vi "Array-Speedtest.vi"() -> ()   [LabVIEW 2016]
uses:
  <userlib>/_OpenG.lib/lvdata/lvdata.llb/Type Descriptor__ogtk.ctl
  <userlib>/_OpenG.lib/lvdata/lvdata.llb/Type Descriptor Header__ogtk.ctl
  <userlib>/_OpenG.lib/lvdata/lvdata.llb/Type Descriptor Enumeration__ogtk.ctl
  SubVis/msgpack_config.ctl
  SubVis/cluster_conversion.ctl
  SubVis/enum_conversion.ctl
  MsgPack.lvlib
  EncodeTypes/enc_a_I8.vi
  EncodeTypes/enc_a_U16.vi
  EncodeTypes/enc_a_I32.vi
  EncodeTypes/enc_a_U8.vi
  EncodeTypes/enc_a_I64.vi
  EncodeTypes/enc_a_I16.vi
  EncodeTypes/enc_a_U32.vi
  EncodeTypes/enc_a_U64.vi
panel:
  out "Element Type Descriptor":T1
  out "Numeric 4":i32
  out "N dims 2":u32
  out "time 4":u32
  out "Array 2":u32[](array[numeric])
  out "N dims":u32
  out "Size(s)":u32[](array[numeric])
  out "x = y?":bool
  out "ms/iter 2":dbl
  out "ms/iter 3":dbl
  out "Array Out 2":u8[](array[numeric]) format="%.0x"
  out "Array Out":u8[](array[numeric]) format="%.0x"
  out "Numeric 3":i32
  out "time 3":u32
  out "Array":u32[](array[numeric])
  out "Type Descriptor Header 2":T2 {"type" format="%.0x"}
  out "Type Descriptor 2":T1
  out "Numeric 2":i32
  out "Numeric":i32
  out "time 2":u32
  out "time":u32
  out "Array":u8[](array[numeric]) format="%.0x"
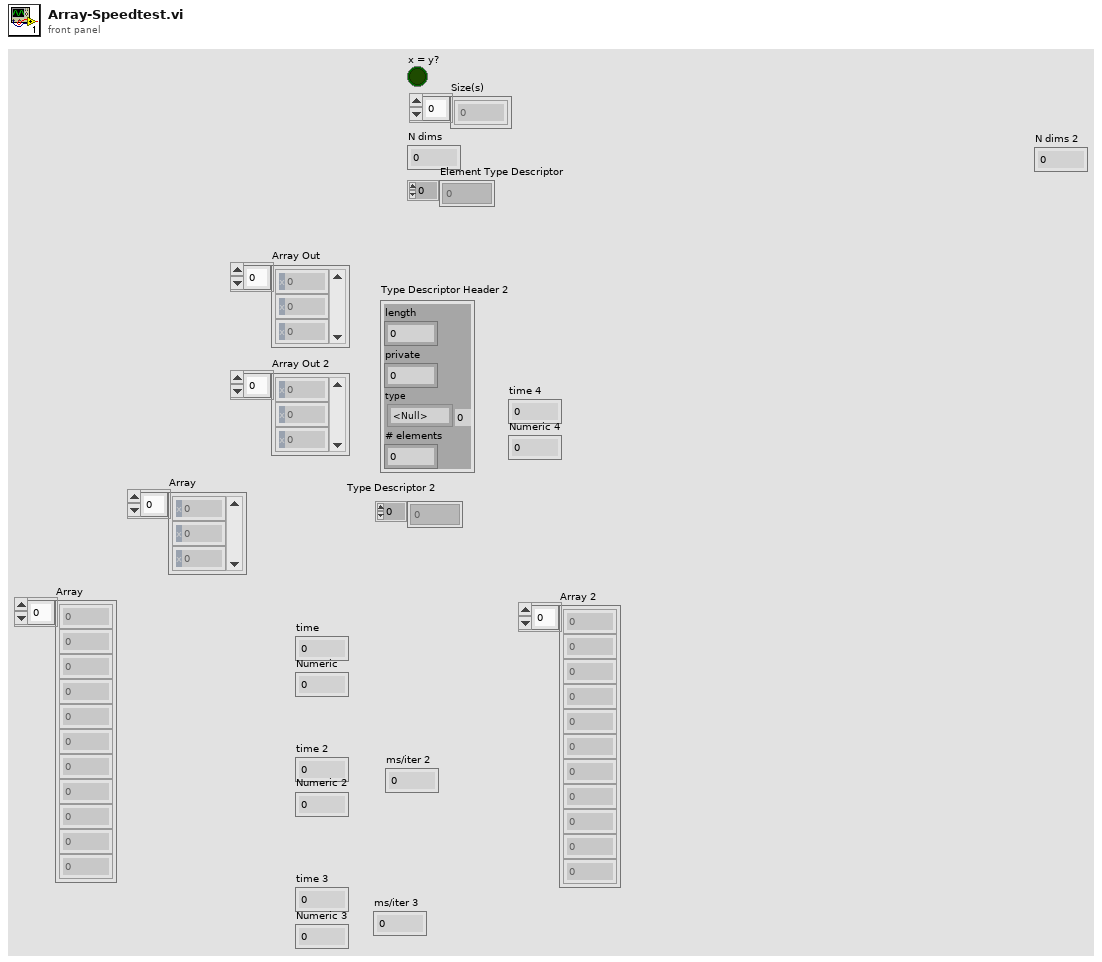
[diagram p1: front panel]
types:
  T1 = typedef "Type Descriptor__ogtk.ctl" = i16[]
  T2 = typedef "Type Descriptor Header__ogtk.ctl" = cluster{"length":u16, "private":u8, "type":T3, "# elements":u16}
  T3 = typedef "Type Descriptor Enumeration__ogtk.ctl" = enum8{"<Null>", "I8", "I16", "I32", "I64", "U8", "U16", "U32", "U64", "SGL", "DBL", "EXT", "CSG", "CDB", "CXT", "0x0F", "0x10", "0x11", "0x12", "0x13", "0x14", "Enum U8", "Enum U16", "Enum U32", "Enum U64", "SGL PQ", "DBL PQ", "EXT PQ", "CSG PQ", "CDB PQ", "CXT PQ", "0x1F", "0x20", "Boolean", "0x22", "0x23", "0x24", "0x25", "0x26", "0x27", "0x28", "0x29", "0x2A", "0x2B", "0x2C", "0x2D", "0x2E", "0x2F", "String", "0x31", "Path", "Pict", "0x34", "0x35", "0x36", "DAQ", "0x38", "0x39", "0x3A", "0x3B", "0x3C", "0x3D", "0x3E", "0x3F", "Array", "0x41", "0x42", "0x43", "0x44", "0x45", "0x46", "0x47", "0x48", "0x49", "0x4A", "0x4B", "0x4C", "0x4D", "0x4E", "0x4F", "Cluster", "0x51", "0x52", "Variant", "Waveform", "0x55", "0x56", "0x57", "0x58", "0x59", "0x5A", "0x5B", "0x5C", "0x5D", "0x5E", "0x5F", "0x60", "0x61", "0x62", "0x63", "0x64", "0x65", "0x66", "0x67", "0x68", "0x69", "0x6A", "0x6B", "0x6C", "0x6D", "0x6E", "0x6F", "Refnum"}
  T4 = typedef "MsgPack.lvlib/msgpack_config.ctl" = cluster{"Cluster Conversion":T5, "Enum Conversion":T6, "Use ArrayType":bool}
  T5 = typedef "MsgPack.lvlib/cluster_conversion.ctl" = enum16{"to map", "to array"}
  T6 = typedef "MsgPack.lvlib/enum_conversion.ctl" = enum16{"to uint", "to string"}
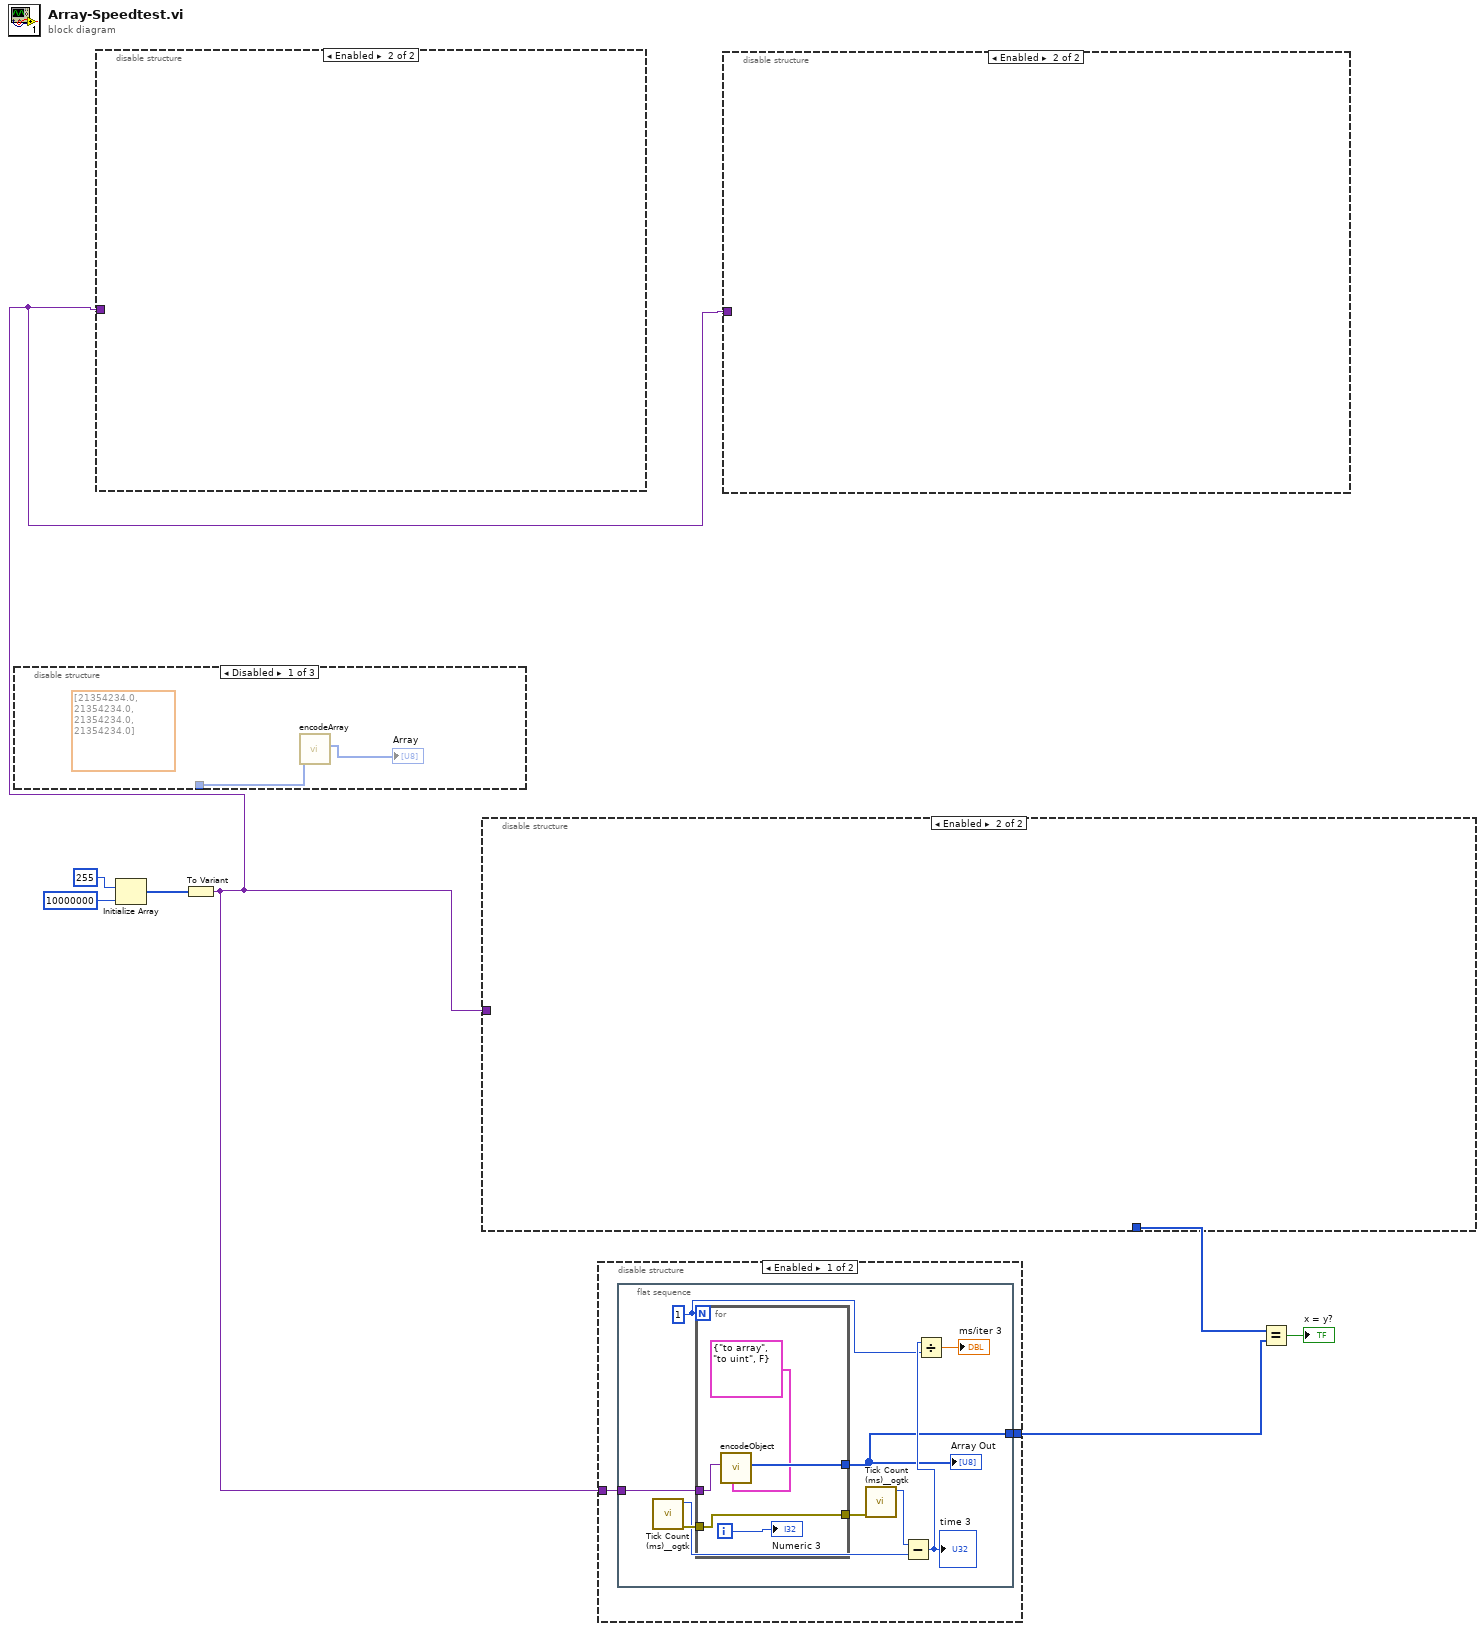
[diagram p0: block diagram]
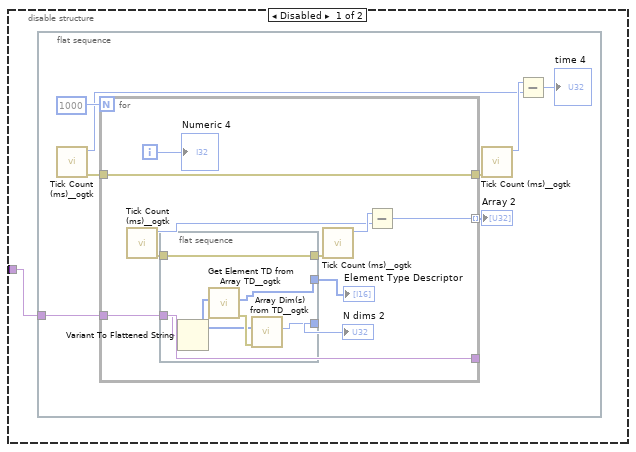
[diagram p2: hidden frame]
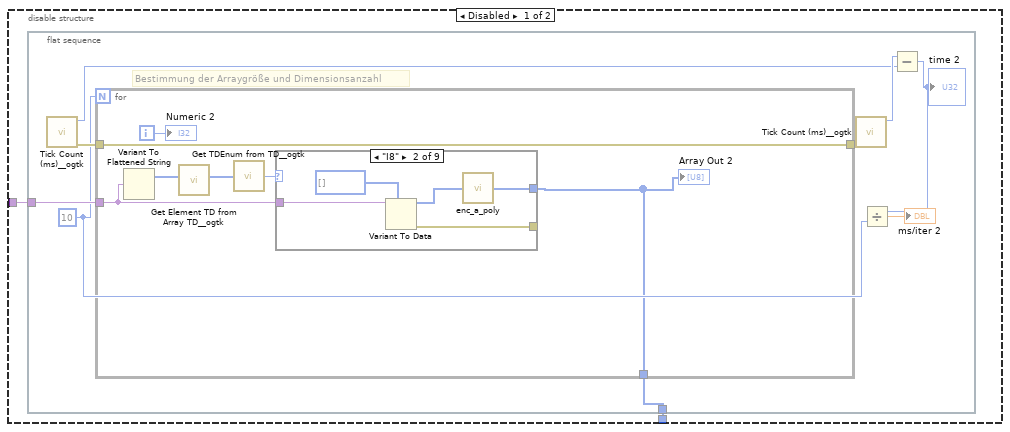
[diagram p4: hidden frame]
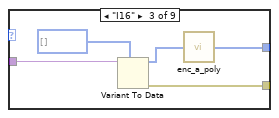
[diagram p6: hidden frame]
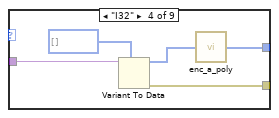
[diagram p7: hidden frame]
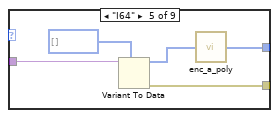
[diagram p8: hidden frame]
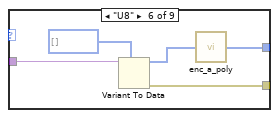
[diagram p9: hidden frame]
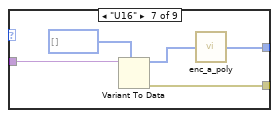
[diagram p10: hidden frame]
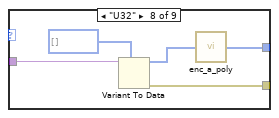
[diagram p11: hidden frame]
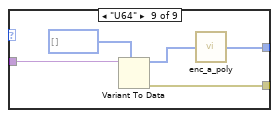
[diagram p12: hidden frame]
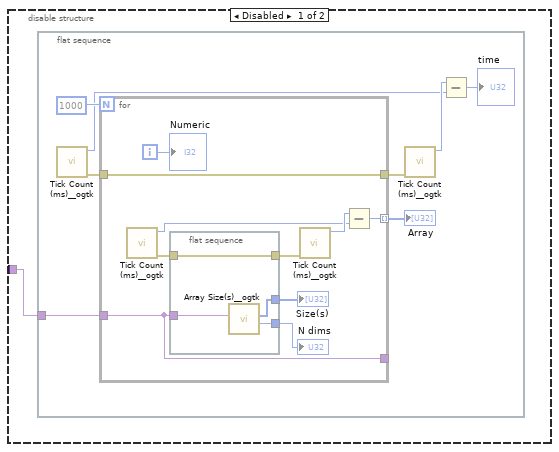
[diagram p13: hidden frame]
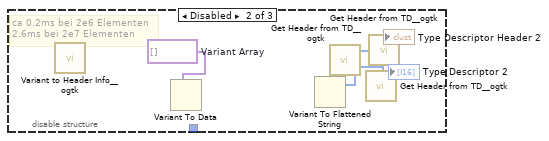
[diagram p14: hidden frame]
diagram:
  n1 = disable-structure shown="Disabled" {
    disable-tunnel: _ -> [w9 _ _]
    frame Disabled {
      (unwired) dbl[] [21354234.0, 21354234.0, 21354234.0, 21354234.0]
      n2 = call "encodeArray.vi"("Variant"=w9) -> ("Array"=→"Array":u8[])  [unwired: 9 in, 1 out]
    }
    frame Disabled {
      w12 = variant[] []  # Variant Array
      # "ca 0.2ms bei 2e6 Elementen\n2.6ms bei 2e7 Elementen"
      n3 = call <userlib>:"Variant to Header Info__ogtk.vi"() -> ()  [unwired: 4 in, 3 out]
      n4 = Variant To Data(type=w12) -> ()  [unwired: 2 in, 2 out]
      n5 = Variant To Flattened String() -> (1:w11:i16[])  [unwired: 1 in, 1 out]
      "Type Descriptor 2" <- w11
      n6 = call <userlib>:"Get Header from TD__ogtk.vi"() -> ()  [unwired: 1 in, 1 out]
      n7 = call <userlib>:"Get Header from TD__ogtk.vi"() -> ()  [unwired: 1 in, 1 out]
      n8 = call <userlib>:"Get Header from TD__ogtk.vi"("Type Descriptor"=w11) -> ("Type Descriptor Header"=→"Type Descriptor Header 2":T2)
    }
    frame Enabled {
    }
  }
  n9 = Initialize Array(u8 255, 10000000 ("dimension size")) -> (w5:u8[])
  n10 = To Variant(anything=w5) -> (Variant=w1:variant)
  n11 = disable-structure shown="Enabled" {
    disable-tunnel: w1 -> [w13 _]
    frame Disabled {
      n12 = flat-sequence {
        tunnel: w13 -> [w15]
        frame #0 {
          n13 = call <userlib>:"Tick Count (ms)__ogtk.vi"() -> ("error out"=w20:errorcluster, "millisecond timer value"=w17:u32)  [unwired: 10 in]
          n14 = for {
            N: 1000 -> [_]
            tunnel: w15 -> [w29]
            tunnel: w20 -> [w31]
            tunnel: [w31] -> w19
            tunnel: [w29] -> _
            tunnel: [w24] -> w14 mode=indexing
            i -> [w30]
            n15 = call <userlib>:"Tick Count (ms)__ogtk.vi"() -> ("error out"=w28:errorcluster, "millisecond timer value"=w25:u32)  [unwired: 10 in]
            n16 = flat-sequence {
              tunnel: w29 -> [w34]
              tunnel: w28 -> [w35]
              tunnel: [w35] -> w27
              tunnel: [w33] -> w23
              tunnel: [w32] -> w22
              frame #0 {
                n17 = call <userlib>:"Array Size(s)__ogtk.vi"("Array"=w34) -> ("N dims"=w32:u32, "Size(s)"=w33:u32[])  [unwired: 8 in, 1 out]
              }
            }
            n18 = call <userlib>:"Tick Count (ms)__ogtk.vi"("error in (no error)"=w27) -> ("millisecond timer value"=w26:u32)  [unwired: 9 in, 1 out]
            n19 = Subtract(x=w26, y=w25) -> (x-y=w24:u32)
            "Numeric" <- w30
            "Size(s)" <- w23
            "N dims" <- w22
          }
          "Array" <- w14
          n20 = call <userlib>:"Tick Count (ms)__ogtk.vi"("error in (no error)"=w19) -> ("millisecond timer value"=w18:u32)  [unwired: 9 in, 1 out]
          n21 = Subtract(x=w18, y=w17) -> (x-y=→"time":u32)
        }
      }
    }
    frame Enabled {
    }
  }
  n22 = disable-structure shown="Enabled" {
    disable-tunnel: w1 -> [w37 _]
    disable-tunnel: [w36 _] -> w4
    frame Disabled {
      n23 = flat-sequence {
        tunnel: w37 -> [w42]
        tunnel: [w38] -> w36
        frame #0 {
          w39 = 10
          # "Bestimmung der Arraygröße und Dimensionsanzahl"
          n24 = call <userlib>:"Tick Count (ms)__ogtk.vi"() -> ("error out"=w46:errorcluster, "millisecond timer value"=w43:u32)  [unwired: 10 in]
          n25 = for {
            N: w39 -> [_]
            tunnel: w42 -> [w51]
            tunnel: w46 -> [w53]
            tunnel: [w53] -> w45
            tunnel: [w47] -> w38
            i -> [w52]
            n26 = Variant To Flattened String(Variant=w51) -> (1:w48:i16[])  [unwired: 1 out]
            n27 = call <userlib>:"Get Element TD from Array TD__ogtk.vi"("Array Type Descriptor"=w48) -> ("Element Type Descriptor"=w50:T1)  [unwired: 9 in, 1 out]
            n28 = call <userlib>:"Get TDEnum from TD__ogtk.vi"("Type Descriptor"=w50) -> ("Type Descriptor Enumeration"=w49:T3)  [unwired: 4 in]
            n29 = case shown="\"I8\"" w49 {
              tunnel: w51 -> [_ w58 w63 w68 w73 w78 w83 w88 w93]
              tunnel: [_ w54 w59 w64 w69 w74 w79 w84 w89] -> w47
              tunnel: [_ w55 w61 w65 w70 w75 w80 w85 w90] -> _
              frame "<Null>", Default {
              }
              frame "I8" {
                n30 = Variant To Data(type=i8[] [], Variant=w58) -> (data=w56:i8[], error out=w55:errorcluster)  [unwired: 1 in]
                n31 = call-poly "enc_a_poly.vi"("Array In"=w56) -> ("Array Out"=w54:u8[])
              }
              frame "I16" {
                n32 = Variant To Data(type=i16[] [], Variant=w63) -> (data=w60:i16[], error out=w61:errorcluster)  [unwired: 1 in]
                n33 = call-poly "enc_a_poly.vi"("Array In"=w60) -> ("Array Out"=w59:u8[])
              }
              frame "I32" {
                n34 = Variant To Data(type=i32[] [], Variant=w68) -> (data=w66:i32[], error out=w65:errorcluster)  [unwired: 1 in]
                n35 = call-poly "enc_a_poly.vi"("Array In"=w66) -> ("Array"=w64:u8[])
              }
              frame "I64" {
                n36 = Variant To Data(type=i64[] [], Variant=w73) -> (data=w71:i64[], error out=w70:errorcluster)  [unwired: 1 in]
                n37 = call-poly "enc_a_poly.vi"("Array In"=w71) -> ("Array Out"=w69:u8[])
              }
              frame "U8" {
                n38 = Variant To Data(type=u8[] [], Variant=w78) -> (data=w76:u8[], error out=w75:errorcluster)  [unwired: 1 in]
                n39 = call-poly "enc_a_poly.vi"("Array In"=w76) -> ("Array Out"=w74:u8[])
              }
              frame "U16" {
                n40 = Variant To Data(type=u16[] [], Variant=w83) -> (data=w81:u16[], error out=w80:errorcluster)  [unwired: 1 in]
                n41 = call-poly "enc_a_poly.vi"("Array In"=w81) -> ("Array Out"=w79:u8[])
              }
              frame "U32" {
                n42 = Variant To Data(type=u32[] [], Variant=w88) -> (data=w86:u32[], error out=w85:errorcluster)  [unwired: 1 in]
                n43 = call-poly "enc_a_poly.vi"("Array In"=w86) -> ("Array Out"=w84:u8[])
              }
              frame "U64" {
                n44 = Variant To Data(type=u64[] [], Variant=w93) -> (data=w91:u64[], error out=w90:errorcluster)  [unwired: 1 in]
                n45 = call-poly "enc_a_poly.vi"("Array In"=w91) -> ("Array Out"=w89:u8[])
              }
            }
            "Array Out 2" <- w47
            "Numeric 2" <- w52
          }
          n46 = call <userlib>:"Tick Count (ms)__ogtk.vi"("error in (no error)"=w45) -> ("millisecond timer value"=w44:u32)  [unwired: 9 in, 1 out]
          n47 = Subtract(x=w44, y=w43) -> (x-y=w40:u32)
          "time 2" <- w40
          n48 = Divide(x=w40, y=w39) -> (x/y=→"ms/iter 2":dbl)
        }
      }
    }
    frame Enabled {
    }
  }
  n49 = disable-structure shown="Enabled" {
    disable-tunnel: w1 -> [w95 _]
    disable-tunnel: [w94 _] -> w3
    frame Enabled {
      n50 = flat-sequence {
        tunnel: w95 -> [w101]
        tunnel: [w96] -> w94
        frame #0 {
          w99 = 1
          n51 = call <userlib>:"Tick Count (ms)__ogtk.vi"() -> ("error out"=w104:errorcluster, "millisecond timer value"=w102:u32)  [unwired: 10 in]
          n52 = for {
            N: w99 -> [_]
            tunnel: w101 -> [w105]
            tunnel: w104 -> [w107]
            tunnel: [w108] -> w96
            tunnel: [w107] -> w97
            i -> [w109]
            n53 = call "encodeObject.vi"("MsgPack Config"=T4 {"Cluster Conversion"=enum."to array", "Enum Conversion"=enum."to uint", "Use ArrayType"=FALSE}, "Variant"=w105) -> ("Array"=w108:u8[])  [unwired: 8 in, 1 out]
            "Numeric 3" <- w109
          }
          "Array Out" <- w96
          n54 = call <userlib>:"Tick Count (ms)__ogtk.vi"("error in (no error)"=w97) -> ("millisecond timer value"=w103:u32)  [unwired: 9 in, 1 out]
          n55 = Subtract(x=w103, y=w102) -> (x-y=w100:u32)
          "time 3" <- w100
          n56 = Divide(x=w100, y=w99) -> (x/y=→"ms/iter 3":dbl)
        }
      }
    }
    frame Disabled {
    }
  }
  n57 = disable-structure shown="Enabled" {
    disable-tunnel: w1 -> [w110 _]
    frame Disabled {
      n58 = flat-sequence {
        tunnel: w110 -> [w112]
        frame #0 {
          n59 = call <userlib>:"Tick Count (ms)__ogtk.vi"() -> ("error out"=w117:errorcluster, "millisecond timer value"=w114:u32)  [unwired: 10 in]
          n60 = for {
            N: 1000 -> [_]
            tunnel: w112 -> [w126]
            tunnel: w117 -> [w128]
            tunnel: [w128] -> w116
            tunnel: [w126] -> _
            tunnel: [w121] -> w111 mode=indexing
            i -> [w127]
            n61 = call <userlib>:"Tick Count (ms)__ogtk.vi"() -> ("error out"=w125:errorcluster, "millisecond timer value"=w122:u32)  [unwired: 10 in]
            n62 = flat-sequence {
              tunnel: w126 -> [w129]
              tunnel: w125 -> [w134]
              tunnel: [w134] -> w124
              tunnel: [w131] -> w120
              tunnel: [w130] -> w119
              frame #0 {
                n63 = Variant To Flattened String(Variant=w129) -> (1:w132:i16[])  [unwired: 1 out]
                n64 = call <userlib>:"Get Element TD from Array TD__ogtk.vi"("Array Type Descriptor"=w132) -> ("error out"=w133:errorcluster, "Element Type Descriptor"=w130:T1)  [unwired: 9 in]
                n65 = call <userlib>:"Array Dim(s) from TD__ogtk.vi"("error in (no error)"=w133, "Array Type Descriptor"=w132) -> ("N dims"=w131:u32)  [unwired: 8 in, 1 out]
              }
            }
            n66 = call <userlib>:"Tick Count (ms)__ogtk.vi"("error in (no error)"=w124) -> ("millisecond timer value"=w123:u32)  [unwired: 9 in, 1 out]
            n67 = Subtract(x=w123, y=w122) -> (x-y=w121:u32)
            "Numeric 4" <- w127
            "N dims 2" <- w120
            "Element Type Descriptor" <- w119
          }
          "Array 2" <- w111
          n68 = call <userlib>:"Tick Count (ms)__ogtk.vi"("error in (no error)"=w116) -> ("millisecond timer value"=w115:u32)  [unwired: 9 in, 1 out]
          n69 = Subtract(x=w115, y=w114) -> (x-y=→"time 4":u32)
        }
      }
    }
    frame Enabled {
    }
  }
  n70 = Equal?(x=w4, y=w3) -> (x = y?=→"x = y?":bool)
